vi "send.vi"(8 "error in (no error)":errorcluster, 9 "topic":string, 10 "message":string, 11 "ActiveMQBroker in":refnum<class "ActiveMQBroker.lvclass">) -> (0 "error out":errorcluster, 3 "ActiveMQBroker out":refnum<class "ActiveMQBroker.lvclass">)   [LabVIEW 2012, in "ActiveMQBroker.lvclass"]
uses:
  ActiveMQBroker.lvclass
  ActiveMQBroker.lvclass/ActiveMQBroker.ctl
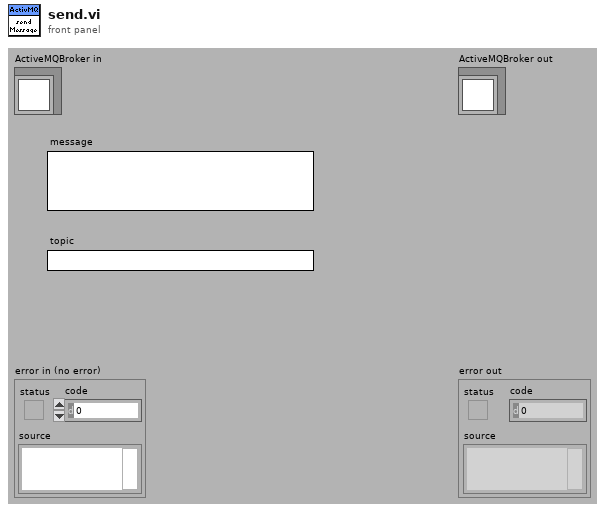
[diagram p1: front panel]
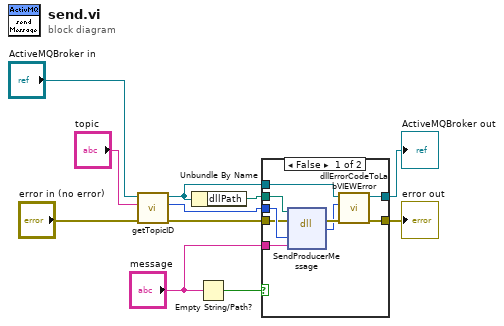
[diagram p0: block diagram]
diagram:
  n1 = call "getTopicID.vi"("error in (no error)"="error in (no error)", "topic"="topic", "ActiveMQBroker in"="ActiveMQBroker in") -> ("error out"=w9:errorcluster, "topicID"=w11:u32, "ActiveMQBroker out"=w6:refnum<class "ActiveMQBroker.lvclass">)  [unwired: 6 in]
  n2 = Unbundle By Name(w6) -> ("dllPath"=w10:path)
  n3 = Empty String/Path?(string/path="message") -> (empty?=w3:bool)
  n4 = case shown="False" w3 {
    tunnel: w11 -> [w20 _]
    tunnel: "message" -> [w19 _]
    tunnel: w10 -> [w18 _]
    tunnel: w9 -> [w17 w21]
    tunnel: [w14 w22] -> w7
    tunnel: w6 -> [w13 w22]
    tunnel: [w12 w21] -> w4
    frame False {
      n5 = dll-call lib="C:/Documents and Settings/dan/My Documents/Lowell/source/DCT/trunk/Components/Common/ActiveMQ/C++ Source/DCTActiveMQWrapper/DCTActiveMQWrapper/Release/DCTActiveMQWrapper.dll" fn="SendProducerMessage"(path in=w18, error in=w17, "ID"=w20, "message"=w19) -> (error out=w16:errorcluster, "return type"=w15:u32)  [unwired: 3 in, 1 out]
      n6 = call "dllErrorCodeToLabVIEWError.vi"("error in (no error)"=w16, "error code in"=w15, "ActiveMQBroker in"=w13) -> ("error out"=w12:errorcluster, "ActiveMQBroker out"=w14:refnum<class "ActiveMQBroker.lvclass">)  [unwired: 7 in]
    }
    frame True {
    }
  }
  "error out" <- w4
  "ActiveMQBroker out" <- w7
